vi "Remove Slot Children.vi"(8 "error in":errorcluster, 11 "slot ref in":T1 format="%.0x") -> (0 "error out":errorcluster, 3 "slot ref out":T1 format="%.0x")   [LabVIEW 2020, in "Scan Engine Scripting.lvlib"]
uses:
  Scan Engine Scripting.lvlib
  <vilib>/NI VeriStand/Custom Device API/Custom Device Item Ref.ctl
  <vilib>/NI VeriStand/Custom Device API/Custom Device API.lvlib
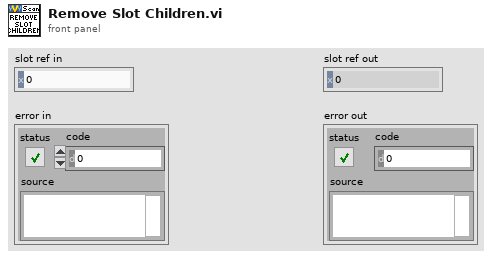
[diagram p1: front panel]
types:
  T1 = typedef "Custom Device API.lvlib/Custom Device Item Ref.ctl" = u64
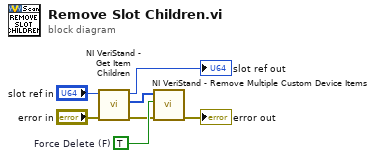
[diagram p0: block diagram]
diagram:
  w3 = TRUE  # Force Delete (F)
  n1 = call <vilib>:"NI VeriStand - Get Item Children.vi"("error in (no error)"="error in", "Item Ref in"="slot ref in") -> ("error out"=w2:errorcluster, "Child Refs"=w1:T1[], "Item Ref out"=→"slot ref out":T1)  [unwired: 6 in, 1 out]
  n2 = call <vilib>:"NI VeriStand - Remove Multiple Custom Device Items.vi"("error in (no error)"=w2, "Force Delete (F)"=w3, "Item Refs in"=w1) -> ("error out"=→"error out":errorcluster)  [unwired: 7 in, 1 out]
